vi "SetParam.vi"(8 "error in (no error)":errorcluster caption="entrée d'erreur (pas d'erreur)", 10 "pairwise_distances_argmin":T1={"axis"=1, "metric "="euclidean", "metric_kwargs"={"metric"=[], "kwargs"=[]}}, 11 "Argmin.lvclass":refnum<class "Argmin.lvclass">) -> (0 "error out":errorcluster caption="sortie d'erreur", 3 "Argmin.lvclass":refnum<class "Argmin.lvclass">)   [LabVIEW 2020, in "Argmin.lvclass"]
doc: "Set Parameters"
uses:
  Argmin.lvclass
  Argmin.lvclass/Argmin.ctl
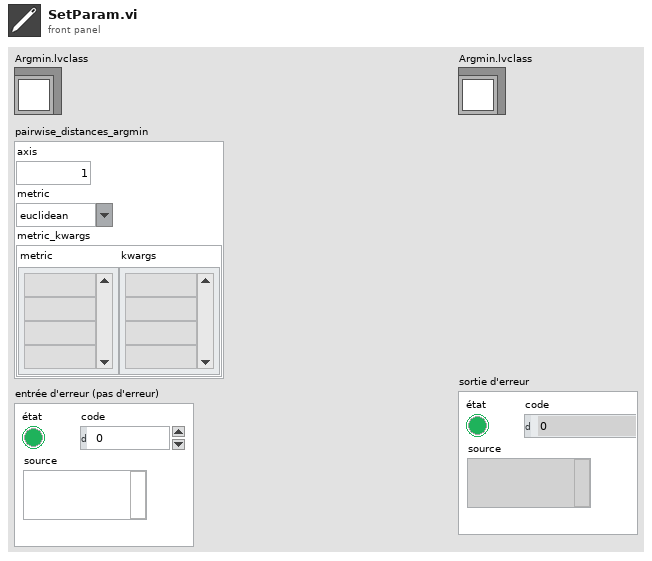
[diagram p1: front panel]
types:
  T1 = cluster{"axis":i32, "metric ":string, "metric_kwargs":cluster{"metric":string[], "kwargs":string[]}}
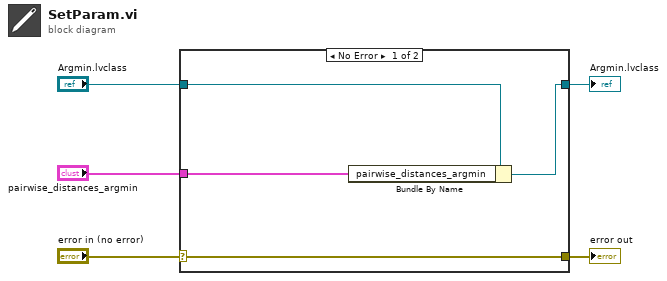
[diagram p0: block diagram]
diagram:
  n1 = case shown="No Error" "error in (no error)" {
    selector: "error in (no error)" -> [w9 w10]
    tunnel: [w9 w10] -> w4
    tunnel: [w7 w11] -> w2
    tunnel: "Argmin.lvclass" -> [w8 w11]
    tunnel: "pairwise_distances_argmin" -> [w6 _]
    frame No Error {
      n2 = Bundle By Name(cluster=w8, "pairwise_distances_argmin"=w6) -> (w7:refnum<class "Argmin.lvclass">)
    }
    frame Error {
    }
  }
  "error out" <- w4
  "Argmin.lvclass" <- w2
